vi "Init.vi"(7 "I2C #":T1=-1, 8 "error in (no error)":errorcluster, 10 "Session In":refnum<class "Session.lvclass">) -> (0 "error out":errorcluster, 3 "AMG8833 8x8 Camera Out":refnum<class "AMG8833 8x8 Camera.lvclass">)   [LabVIEW 2020, in "CTI-Peripheral.lvlib" / "AMG8833 8x8 Camera.lvclass"]
uses:
  AMG8833 8x8 Camera.lvclass
  CTI/Session/Session.lvclass
  CTI/I2C Number.ctl
  CTI/I2C Address.ctl
  CTI/I2C Connection/I2C Connection.lvclass/I2C Connection.ctl
  AMG8833 8x8 Camera.lvclass/AMG8833 8x8 Camera.ctl
  CTI/I2C Connection/I2C Connection.lvclass
  CTI/CTI.lvlib
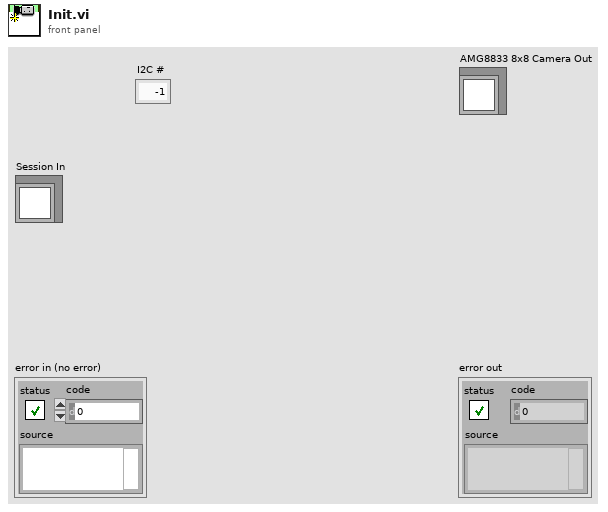
[diagram p1: front panel]
types:
  T1 = typedef "CTI.lvlib/I2C Number.ctl" = i8
  T2 = typedef "CTI.lvlib/I2C Address.ctl" = u8
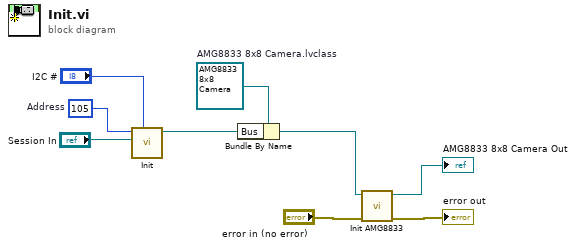
[diagram p0: block diagram]
diagram:
  w5 = refnum<class "AMG8833 8x8 Camera.lvclass"> refnum  # AMG8833 8x8 Camera.lvclass
  w6 = T2 105  # Address
  n1 = call "Init.vi"("I2C #"="I2C #", "Session"="Session In", "Address"=w6) -> ("I2C Connection"=w9:refnum<class "I2C Connection.lvclass">)  [unwired: 7 in, 1 out]
  n2 = Bundle By Name(cluster=w5, "Bus"=w9) -> (w4:refnum<class "AMG8833 8x8 Camera.lvclass">)
  n3 = call "Init AMG8833.vi"("error in (no error)"="error in (no error)", "AMG8833 8x8 Camera in"=w4) -> ("error out"=→"error out":errorcluster, "AMG8833 8x8 Camera out"=→"AMG8833 8x8 Camera Out":refnum<class "AMG8833 8x8 Camera.lvclass">)  [unwired: 8 in]
